vi "Tetrix_Motor_Test.vi"() -> ()   [LabVIEW 2013]
uses:
  <userlib>/KNR OS 3.0 LabVIEW Toolkit/support SubVI/_Controls/Lego Port.ctl
panel:
  in  "DC Motor ID(110)":u32=210
  in  "Move":cluster{"Pcmd":i32, "Vcmd":i32}={"Pcmd"=-40, "Vcmd"=400}
  out "電壓":dbl
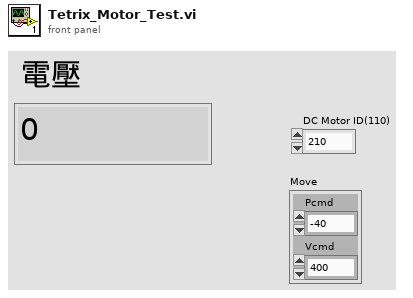
[diagram p1: front panel]
types:
  T1 = typedef "Lego Port.ctl" = enum8{"L1", "LS1", "LS3", "LS4", "LS2"}
  T2 = typedef "KNR3 Reference.ctl" = cluster{"FPGA Session":refnum<class "FPGA Interface Base.lvclass">, "Resource":T3}
  T3 = typedef "Resource.ctl" = enum16{"KNRm_DDRC", "KNRm_DDDD", "KNRm_DDDR", "KNRm_DDDC", "KNR"}
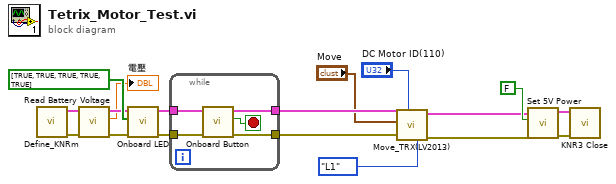
[diagram p0: block diagram]
diagram:
  n1 = call "Define_KNRm.vi"() -> ("error out"=w17:errorcluster, "KNR out"=w18:T2)  [unwired: 10 in]
  n2 = call <userlib>:"Read Battery Voltage.vi"("error in (no error)"=w17, "KNR in"=w18) -> ("error out"=w14:errorcluster, "Voltage"=→"電壓":dbl, "KNR out"=w15:T2)  [unwired: 7 in]
  n3 = call <userlib>:"Onboard LED.vi"("error in (no error)"=w14, "LED List"=bool[] [TRUE, TRUE, TRUE, TRUE, TRUE], "KNR in"=w15) -> ("error out"=w8:errorcluster, "KNR out"=w9:T2)  [unwired: 7 in]
  n4 = while {
    tunnel: [w23] -> w6
    tunnel: w9 -> [w22]
    tunnel: [w20] -> w7
    tunnel: w8 -> [w19]
    stop <- w21 stop-if-true
    n5 = call <userlib>:"Onboard Button.vi"("error in (no error)"=w19, "KNR in"=w22) -> ("error out"=w23:errorcluster, "value"=w21:bool, "KNR out"=w20:T2)  [unwired: 7 in]
  }
  n6 = call "Move_TRX(LV2013).vi"("DC Motor ID(110)"="DC Motor ID(110)", "error in"=w6, "Port (LS1)"=Lego_Port."L1", "Move"="Move", "KNR in"=w7) -> ("error out"=w4:errorcluster, "KNR out"=w5:T2)  [unwired: 5 in]
  n7 = call <userlib>:"Set 5V Power.vi"("error in (no error)"=w4, "5V Power(T)"=FALSE, "KNR in"=w5) -> ("error out"=w12:errorcluster, "KNR out"=w11:T2)  [unwired: 7 in]
  n8 = call <userlib>:"KNR3 Close.vi"("error in (no error)"=w12, "KNR in"=w11) -> ()  [unwired: 9 in, 1 out]
